vi "Quotes.vi"(7 "Action":enum8{"Escape", "Unescape"}(ring), 10 "Is String? (T)":bool=TRUE, 11 "String in":string) -> (3 "String out":string)   [LabVIEW 2018, in "Config.lvlib"]
uses:
  Config.lvlib
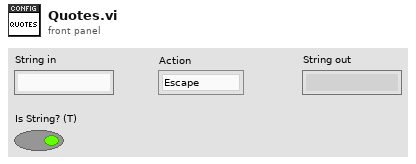
[diagram p1: front panel]
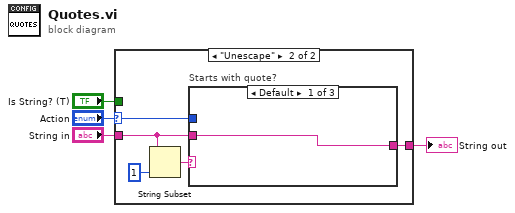
[diagram p0: block diagram]
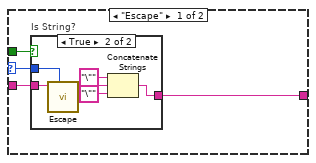
[diagram p2: hidden frame]
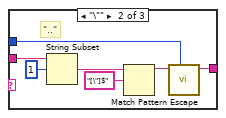
[diagram p4: hidden frame]
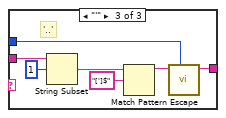
[diagram p5: hidden frame]
diagram:
  n1 = case shown="\"Unescape\"" "Action" {
    selector: "Action" -> [w7 w17]
    tunnel: "String in" -> [w8 w18]
    tunnel: [w6 w16] -> w2
    tunnel: "Is String? (T)" -> [w5 _]
    frame "Escape" {
      n2 = case "Is String?" shown="True" w5 {
        tunnel: w8 -> [w9 w15]
        tunnel: w7 -> [_ w14]
        tunnel: [w9 w12] -> w6
        frame False {
        }
        frame True {
          n3 = call "Escape.vi"("Action"=w14, "String in"=w15) -> ("String out"=w13:string)  [unwired: 8 in, 1 out]
          n4 = Concatenate Strings("\"" ("string"), w13, "\"" ("string")) -> (w12:string)
        }
      }
    }
    frame "Unescape" {
      n5 = String Subset(string=w18, length (rest)=1 ("length (rest)")) -> (substring=w19:string)  [unwired: 1 in]
      n6 = case "Starts with quote?" shown="Default" w19 {
        tunnel: w18 -> [w21 w28 w35]
        tunnel: w17 -> [_ w23 w30]
        tunnel: [w21 w22 w29] -> w16
        frame Default {
        }
        frame "\"" {
          # "\"..\""
          n7 = String Subset(string=w28, offset (0)=1) -> (substring=w26:string)  [unwired: 1 in]
          n8 = Match Pattern(string=w26, regular expression="[\"]$") -> (before substring=w24:string)  [unwired: 1 in, 3 out]
          n9 = call "Escape.vi"("Action"=w23, "String in"=w24) -> ("String out"=w22:string)  [unwired: 8 in, 1 out]
        }
        frame "'" {
          # "'..'"
          n10 = String Subset(string=w35, offset (0)=1) -> (substring=w33:string)  [unwired: 1 in]
          n11 = Match Pattern(string=w33, regular expression="[']$") -> (before substring=w31:string)  [unwired: 1 in, 3 out]
          n12 = call "Escape.vi"("Action"=w30, "String in"=w31) -> ("String out"=w29:string)  [unwired: 8 in, 1 out]
        }
      }
    }
  }
  "String out" <- w2
